vi "ScannedNodeDatabaseEditor.vi"() -> ()   [LabVIEW 2022 SP3]
uses:
  ScannedNodeArray.ctl
  LymphNodeInfo.ctl
  TissueTypeScan.ctl
panel:
  in  "stop":bool
  in  "Previously Scanned Nodes":T1 {"Year" format="%02d"; "Patient Number" format="%03d"; "Node Number" format="%02d"}
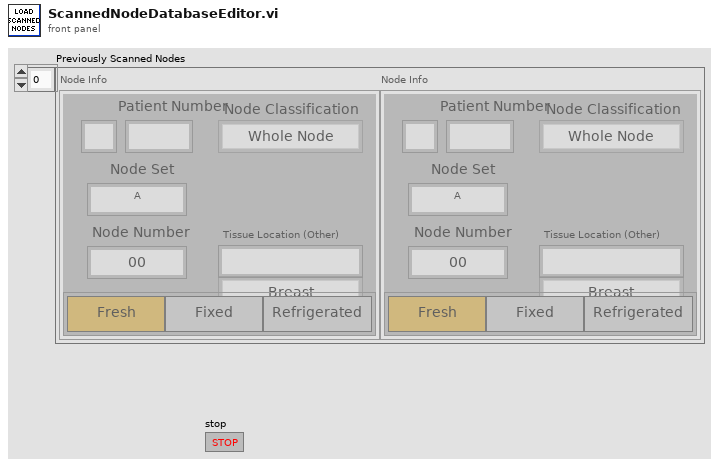
[diagram p1: front panel]
types:
  T1 = typedef "ScannedNodeArray.ctl" = T2[]
  T2 = typedef "LymphNodeInfo.ctl" = cluster{"Patient Number":u32, "Node Set":string, "Node Number":u32, "Tissue Type":T3, "Tissue Location (Other)":string, "Node Classification":enum16{"Whole Node", "Piece A", "Piece B", "Piece C"}, "Fresh?":enum32{"Fresh?", "Fixed?", "Refrigerated?"}, "Year":u32}
  T3 = typedef "TissueTypeScan.ctl" = enum16{"Breast", "Gastric", "Stomach", "Rectal", "Colon", "Head & Neck", "Other"}
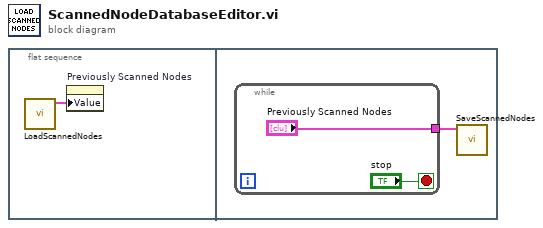
[diagram p0: block diagram]
diagram:
  n1 = flat-sequence {
    frame #0 {
      n2 = call "LoadScannedNodes.vi"() -> ("Previously Scanned Nodes"=w1:T1)  [unwired: 11 in]
      n3 = property on="Previously Scanned Nodes" class="Arr (strict)"("Value"=w1) -> ()  [unwired: 2 in, 2 out]
    }
    frame #1 {
      n4 = while {
        tunnel: ["Previously Scanned Nodes"] -> w2
        stop <- "stop" stop-if-true
      }
      n5 = call "SaveScannedNodes.vi"("Scanned Nodes"=w2) -> ()  [unwired: 11 in]
    }
  }
